vi "WHILELOOPandcase.vi"() -> ()   [LabVIEW 2019]
uses:
  <vilib>/measure/NI_MABase.lvlib
panel:
  out "Waveform Graph 4":waveform(dbl)(graph)
  in  "FREQ 4":dbl(knob) scale=0.0..10.0
  out "Waveform Graph 3":dbl[](graph)
  in  "FREQ 3":dbl(knob) scale=0.0..10.0
  in  "index":i32
  in  "FREQ 2":dbl(knob) scale=0.0..10.0
  out "Waveform Graph 2":waveform(dbl)(graph)
  out "ANS":dbl
  in  "b":dbl
  in  "a":dbl
  out "Waveform Graph":waveform(dbl)(graph)
  in  "FREQ":dbl(knob) scale=0.0..10.0
  in  "Enum 2":enum16{"SINE", "COS", "SUR", "TRI", "SAW"}(ring)
  in  "Enum":enum16{"ADD", "SUB", "DIV", "MUP"}(ring)
  out "String 4":string
  in  "String 3":string
  out "String 2":string
  in  "Boolean":bool
  out "String":string
  out "Numeric 3":i32
  out "Numeric 2":i32
  out "Numeric":i32
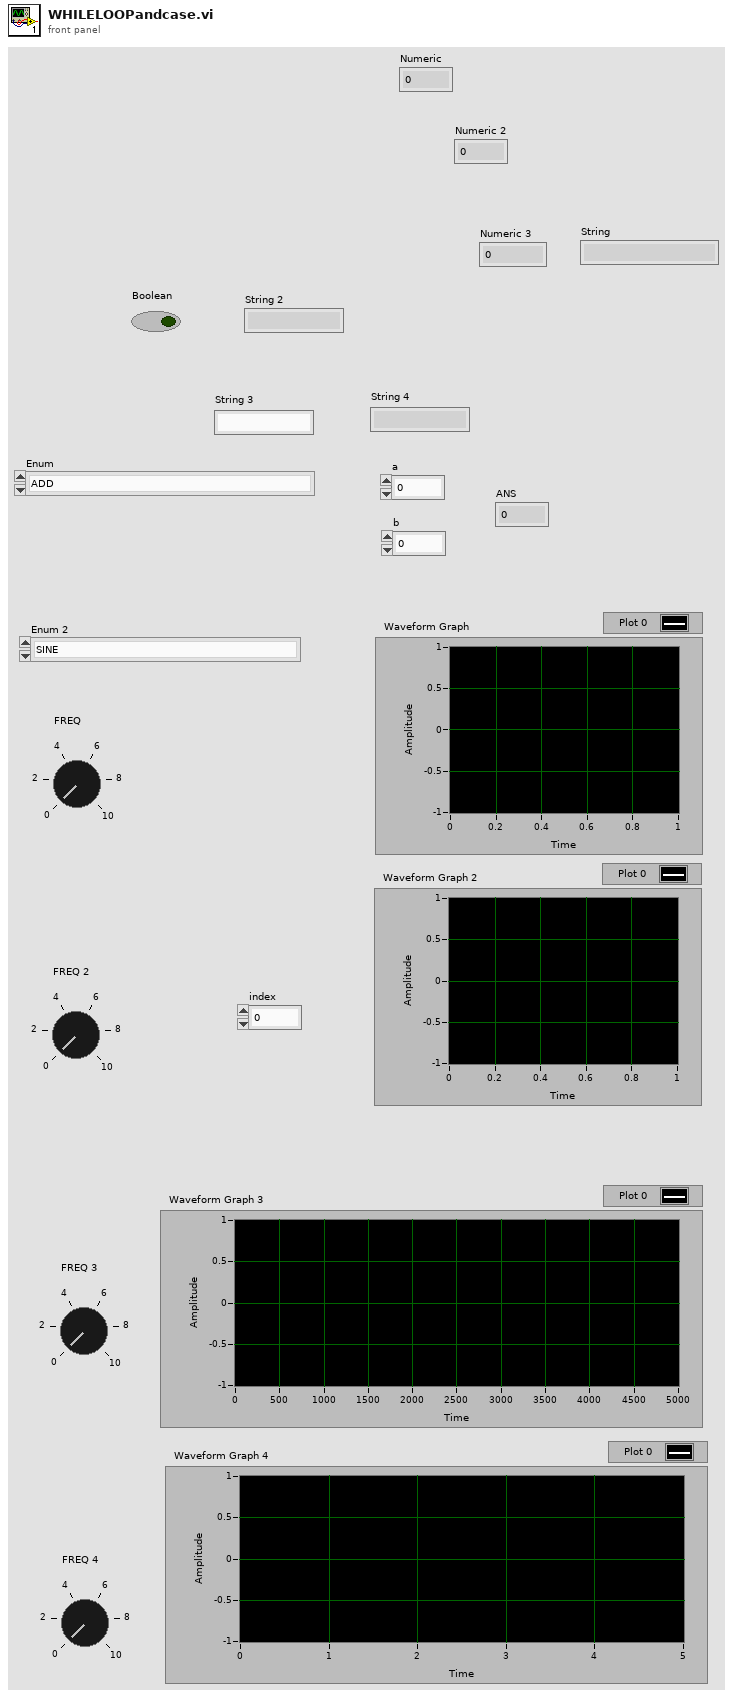
[diagram p1: front panel]
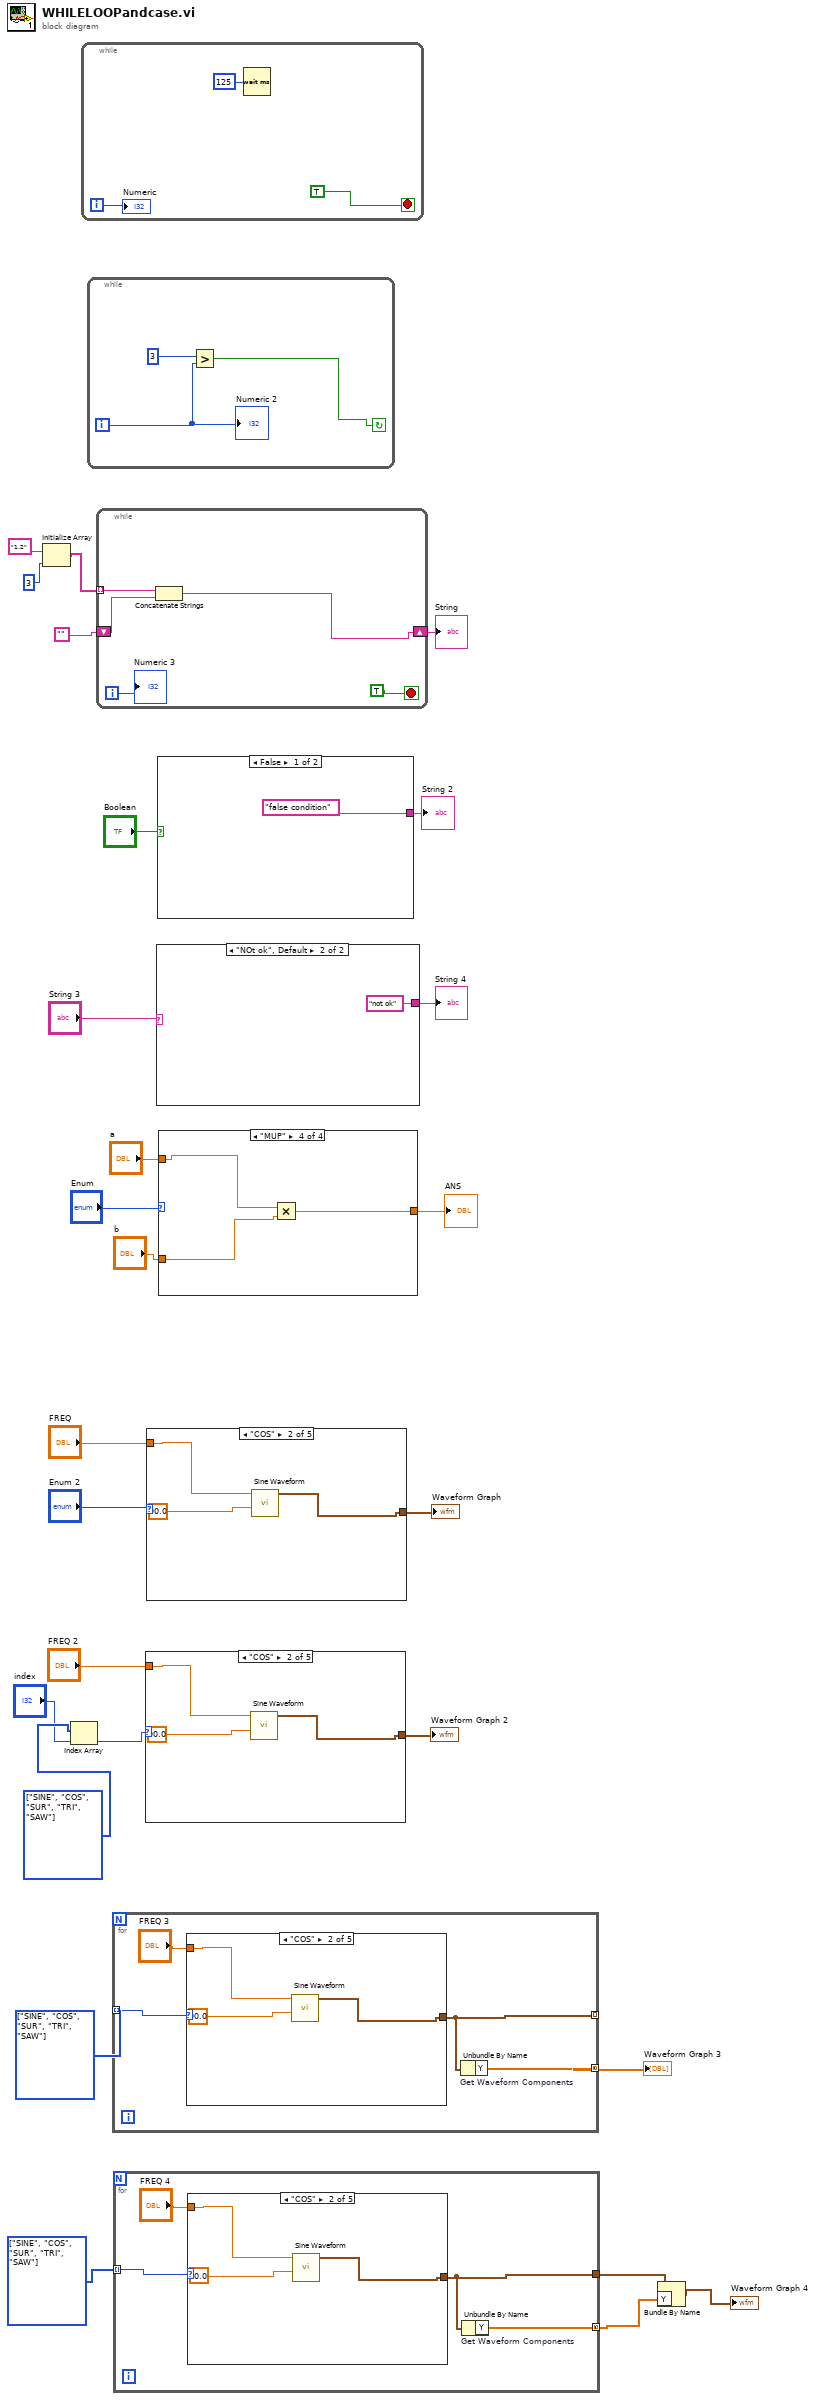
[diagram p0: block diagram]
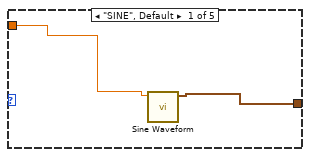
[diagram p2: hidden frame]
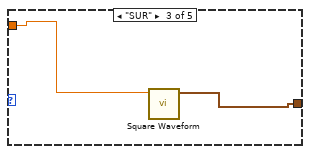
[diagram p3: hidden frame]
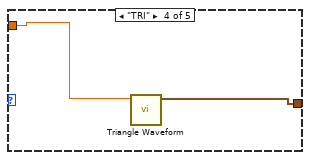
[diagram p4: hidden frame]
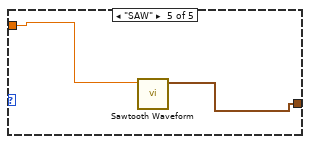
[diagram p5: hidden frame]
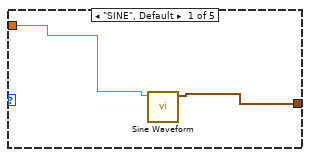
[diagram p6: hidden frame]
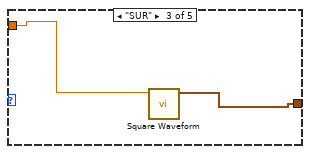
[diagram p7: hidden frame]
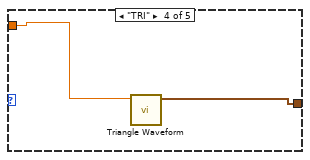
[diagram p8: hidden frame]
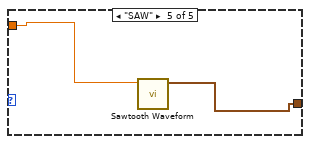
[diagram p9: hidden frame]
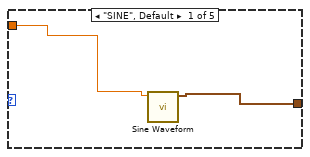
[diagram p10: hidden frame]
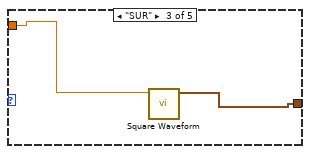
[diagram p11: hidden frame]
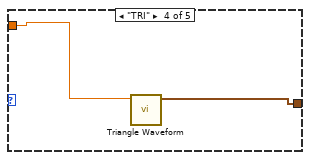
[diagram p12: hidden frame]
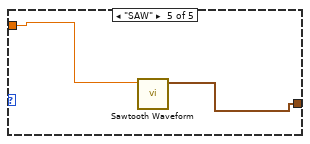
[diagram p13: hidden frame]
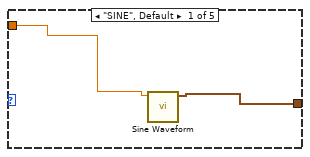
[diagram p14: hidden frame]
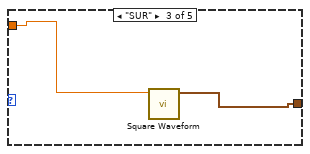
[diagram p15: hidden frame]
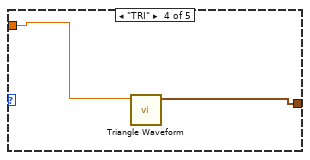
[diagram p16: hidden frame]
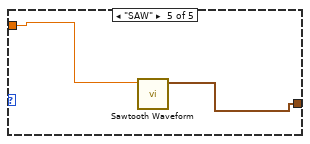
[diagram p17: hidden frame]
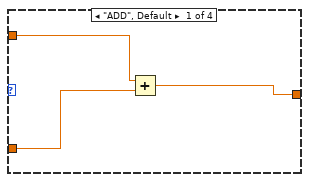
[diagram p18: hidden frame]
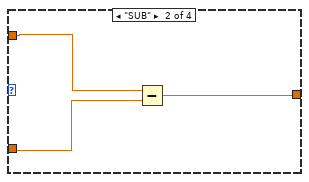
[diagram p19: hidden frame]
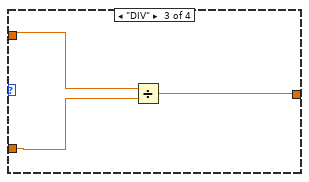
[diagram p20: hidden frame]
diagram:
  w4 = enum16{"SINE", "COS", "SUR", "TRI", "SAW"}[] [enum."SINE", enum."COS", enum."SUR", enum."TRI", enum."SAW"] items=["SINE", "COS", "SUR", "TRI", "SAW"]
  w6 = enum16{"SINE", "COS", "SUR", "TRI", "SAW"}[] [enum."SINE", enum."COS", enum."SUR", enum."TRI", enum."SAW"] items=["SINE", "COS", "SUR", "TRI", "SAW"]
  w9 = enum16{"SINE", "COS", "SUR", "TRI", "SAW"}[] [enum."SINE", enum."COS", enum."SUR", enum."TRI", enum."SAW"] items=["SINE", "COS", "SUR", "TRI", "SAW"]
  n1 = Initialize Array "Initialize Array"("1.2", 3 ("dimension size")) -> (w24:string[])
  n2 = Index Array(array=w9, index="index") -> (element=w8:enum16{"SINE", "COS", "SUR", "TRI", "SAW"})
  n3 = while {
    i -> [w30]
    stop <- TRUE stop-if-true
    n4 = Wait (ms)(milliseconds to wait=u32 125) -> ()  [unwired: 1 out]
    "Numeric" <- w30
  }
  n5 = while {
    i -> [w33]
    stop <- w32 continue-if-true
    n6 = Greater?(x=3, y=w33) -> (0:w32:bool)
    "Numeric 2" <- w33
  }
  n7 = while {
    shift-right: [w35] -> w23
    shift-left: "" -> [w37]
    tunnel: w24 -> [w36] mode=indexing
    i -> [w38]
    stop <- TRUE stop-if-true
    n8 = Concatenate Strings(w36, w37) -> (w35:string)
    "Numeric 3" <- w38
  }
  "String" <- w23
  n9 = for {
    tunnel: w6 -> [w41] mode=indexing
    tunnel: [w40] -> w5 mode=concatenating
    tunnel: [w39] -> _ mode=indexing
    n10 = case shown="\"COS\"" w41 {
      tunnel: "FREQ 3" -> [w44 w47 w49 w51 w53]
      tunnel: [w43 w45 w48 w50 w52] -> w39
      frame "SINE", Default {
        n11 = call <vilib>:"Sine Waveform.vi"("frequency"=w44) -> ("signal out"=w43:waveform(dbl))  [unwired: 9 in, 1 out]
      }
      frame "COS" {
        n12 = call <vilib>:"Sine Waveform.vi"("phase"=90.0, "frequency"=w47) -> ("signal out"=w45:waveform(dbl))  [unwired: 8 in, 1 out]
      }
      frame "SUR" {
        n13 = call <vilib>:"Square Waveform.vi"("frequency"=w49) -> ("signal out"=w48:waveform(dbl))  [unwired: 9 in, 1 out]
      }
      frame "TRI" {
        n14 = call <vilib>:"Triangle Waveform.vi"("frequency"=w51) -> ("signal out"=w50:waveform(dbl))  [unwired: 9 in, 1 out]
      }
      frame "SAW" {
        n15 = call <vilib>:"Sawtooth Waveform.vi"("frequency"=w53) -> ("signal out"=w52:waveform(dbl))  [unwired: 9 in, 1 out]
      }
    }
    n16 = Unbundle By Name "Get Waveform Components"(w39) -> ("Y"=w40:dbl[])
  }
  "Waveform Graph 3" <- w5
  n17 = for {
    tunnel: w4 -> [w56] mode=indexing
    tunnel: [w55] -> w2 mode=concatenating
    tunnel: [w54] -> w3
    n18 = case shown="\"COS\"" w56 {
      tunnel: "FREQ 4" -> [w59 w62 w64 w66 w68]
      tunnel: [w58 w60 w63 w65 w67] -> w54
      frame "SINE", Default {
        n19 = call <vilib>:"Sine Waveform.vi"("frequency"=w59) -> ("signal out"=w58:waveform(dbl))  [unwired: 9 in, 1 out]
      }
      frame "COS" {
        n20 = call <vilib>:"Sine Waveform.vi"("phase"=90.0, "frequency"=w62) -> ("signal out"=w60:waveform(dbl))  [unwired: 8 in, 1 out]
      }
      frame "SUR" {
        n21 = call <vilib>:"Square Waveform.vi"("frequency"=w64) -> ("signal out"=w63:waveform(dbl))  [unwired: 9 in, 1 out]
      }
      frame "TRI" {
        n22 = call <vilib>:"Triangle Waveform.vi"("frequency"=w66) -> ("signal out"=w65:waveform(dbl))  [unwired: 9 in, 1 out]
      }
      frame "SAW" {
        n23 = call <vilib>:"Sawtooth Waveform.vi"("frequency"=w68) -> ("signal out"=w67:waveform(dbl))  [unwired: 9 in, 1 out]
      }
    }
    n24 = Unbundle By Name "Get Waveform Components"(w54) -> ("Y"=w55:dbl[])
  }
  n25 = case shown="\"COS\"" w8 {
    tunnel: "FREQ 2" -> [w70 w73 w75 w77 w79]
    tunnel: [w69 w71 w74 w76 w78] -> w11
    frame "SINE", Default {
      n26 = call <vilib>:"Sine Waveform.vi"("frequency"=w70) -> ("signal out"=w69:waveform(dbl))  [unwired: 9 in, 1 out]
    }
    frame "COS" {
      n27 = call <vilib>:"Sine Waveform.vi"("phase"=90.0, "frequency"=w73) -> ("signal out"=w71:waveform(dbl))  [unwired: 8 in, 1 out]
    }
    frame "SUR" {
      n28 = call <vilib>:"Square Waveform.vi"("frequency"=w75) -> ("signal out"=w74:waveform(dbl))  [unwired: 9 in, 1 out]
    }
    frame "TRI" {
      n29 = call <vilib>:"Triangle Waveform.vi"("frequency"=w77) -> ("signal out"=w76:waveform(dbl))  [unwired: 9 in, 1 out]
    }
    frame "SAW" {
      n30 = call <vilib>:"Sawtooth Waveform.vi"("frequency"=w79) -> ("signal out"=w78:waveform(dbl))  [unwired: 9 in, 1 out]
    }
  }
  "Waveform Graph 2" <- w11
  n31 = case shown="\"COS\"" "Enum 2" {
    tunnel: "FREQ" -> [w81 w84 w86 w88 w90]
    tunnel: [w80 w82 w85 w87 w89] -> w15
    frame "SINE", Default {
      n32 = call <vilib>:"Sine Waveform.vi"("frequency"=w81) -> ("signal out"=w80:waveform(dbl))  [unwired: 9 in, 1 out]
    }
    frame "COS" {
      n33 = call <vilib>:"Sine Waveform.vi"("phase"=90.0, "frequency"=w84) -> ("signal out"=w82:waveform(dbl))  [unwired: 8 in, 1 out]
    }
    frame "SUR" {
      n34 = call <vilib>:"Square Waveform.vi"("frequency"=w86) -> ("signal out"=w85:waveform(dbl))  [unwired: 9 in, 1 out]
    }
    frame "TRI" {
      n35 = call <vilib>:"Triangle Waveform.vi"("frequency"=w88) -> ("signal out"=w87:waveform(dbl))  [unwired: 9 in, 1 out]
    }
    frame "SAW" {
      n36 = call <vilib>:"Sawtooth Waveform.vi"("frequency"=w90) -> ("signal out"=w89:waveform(dbl))  [unwired: 9 in, 1 out]
    }
  }
  "Waveform Graph" <- w15
  n37 = case shown="\"NOt ok\", Default" "String 3" {
    tunnel: ["ok" "not ok"] -> w19
    frame "ok" {
    }
    frame "NOt ok", Default {
    }
  }
  "String 4" <- w19
  n38 = case shown="False" "Boolean" {
    tunnel: ["false condition" "true condition"] -> w21
    frame False {
    }
    frame True {
    }
  }
  "String 2" <- w21
  n39 = case shown="\"MUP\"" "Enum" {
    tunnel: "a" -> [w97 w100 w103 w106]
    tunnel: "b" -> [w96 w99 w101 w105]
    tunnel: [w95 w98 w102 w104] -> w12
    frame "ADD", Default {
      n40 = Add(x=w97, y=w96) -> (x+y=w95:dbl)
    }
    frame "SUB" {
      n41 = Subtract(x=w100, y=w99) -> (x-y=w98:dbl)
    }
    frame "DIV" {
      n42 = Divide(x=w103, y=w101) -> (x/y=w102:dbl)
    }
    frame "MUP" {
      n43 = Multiply(x=w106, y=w105) -> (x*y=w104:dbl)
    }
  }
  "ANS" <- w12
  n44 = Bundle By Name(cluster=w3, "Y"=w2) -> (→"Waveform Graph 4":waveform(dbl))
